vi "read_attributes.vi"(8 "error in (no error)":errorcluster, 11 "OrthogonalMatchingPursuit in":refnum<class "OrthogonalMatchingPursuit.lvclass">) -> (0 "error out":errorcluster, 2 "attributes":T1, 3 "OrthogonalMatchingPursuit out":refnum<class "OrthogonalMatchingPursuit.lvclass">)   [LabVIEW 2020, in "OrthogonalMatchingPursuit.lvclass"]
uses:
  OrthogonalMatchingPursuit.lvclass
  Controls/orthogonal_matching_pursuit_attributes.ctl
  OrthogonalMatchingPursuit.lvclass/OrthogonalMatchingPursuit.ctl
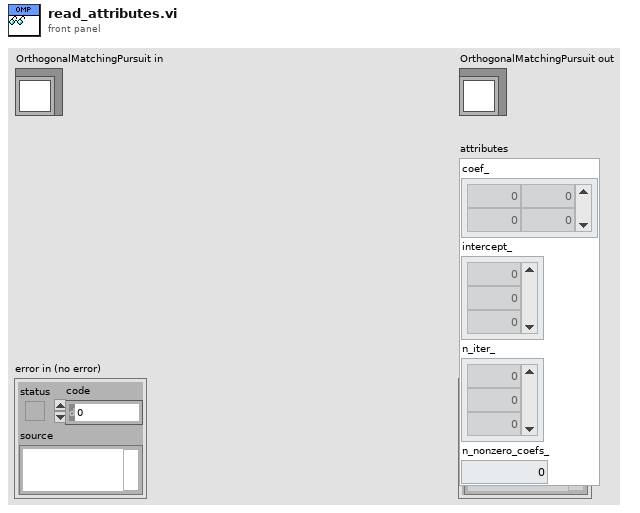
[diagram p1: front panel]
types:
  T1 = typedef "orthogonal_matching_pursuit_attributes.ctl" = cluster{"coef_":dbl[][], "intercept_":dbl[], "n_iter_":dbl[], "n_nonzero_coefs_":dbl}
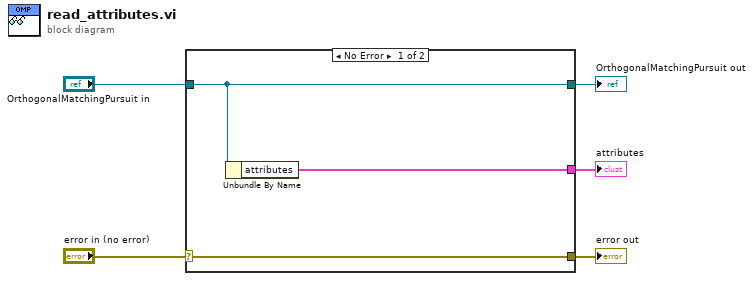
[diagram p0: block diagram]
diagram:
  n1 = case shown="No Error" "error in (no error)" {
    selector: "error in (no error)" -> [w8 w9]
    tunnel: [w8 w9] -> w4
    tunnel: [w7 w10] -> w2
    tunnel: "OrthogonalMatchingPursuit in" -> [w7 w10]
    tunnel: [w6 _] -> w1
    frame No Error {
      n2 = Unbundle By Name(w7) -> ("attributes"=w6:T1)
    }
    frame Error {
    }
  }
  "error out" <- w4
  "OrthogonalMatchingPursuit out" <- w2
  "attributes" <- w1
